vi "PSLDAQ_Read.vi"(4 "Handle In":T1) -> (0 "Int16 Ch2 Data":i16[](array[numeric]), 1 "# Read":i32, 2 "CH2 Data":dbl[](graph), 3 "Int16 Ch1 Data":i16[](array[numeric]), 5 "CH1 Data":dbl[](graph))   [LabVIEW 2010]
doc: "1. 설명\n a. 획득된 데이터를 읽음\n\n2. 기능\n a. PSL-DAQ 장치에서 획득된 2채널의 데이터를 읽음\n \n3. 터미널\n a. 터미널 입력\n ○ Handle In : 장치 핸들\n \n b. 터미널 출력\n ○ Chn Data(n=1~2) : 2채널의 각 채널별 double형 배열 데이터\n ○ Int16 Chn Data(n=1~2) : 2채널의 각 채널별 16bit 부호있는 정수형 배열 데이터\n - PSL-DAQ장치의 ADC 값임. 필요시 데이터 수신 오류 등을 판단할 때 사용 \n ○ #Read : 배열 데이터의 배열의 크기. VI가 호출될 때 읽은 데이터 샘플 수를 의미\n\n4. 주의\n a. PSL DAQ 장치와 통신 연결된 경우에 정상적으로 동작함.\n b. PSLDAQ_AcquireStart 함수가 먼저 호출되어야 함."
uses:
  PSLDAQ_Dll.dll
panel:
  out "# Total Read Num":i32
  # "PSLDAQ_Read\n\n1. 설명\n  a. 획득된 데이터를 읽음\n\n2. 기능\n  a. PSL-DAQ 장치에서 획득된 2채널의 데이터를 읽음\n      \n3. 터미널\n  a. 터미널 입력\n     ○ Handle In : 장치 핸들\n \n  b. 터미널 출력\n     ○ Chn Data(n=1~2) : 2채널의 각 채널별 double형 배열 데이터\n     ○ Int16 Chn Data(n=1~2) : 2채널의 각 채널별 16bit 부호있는 정수형 배열 데이터\n         - PSL-DAQ장치의 ADC 값임. 필요시 데이터 수신 오류 등을 판단할 때 사용 \n     ○ #Read : 배열 데이터의 배열의 크기. VI가 호출될 때 읽은 데이터 샘플 수를 의미\n\n4. 주의\n  a. PSL DAQ 장치와 통신 연결된 경우에 정상적으로 동작함.\n  b. PSLDAQ_AcquireStart 함수가 먼저 호출되어야 함."
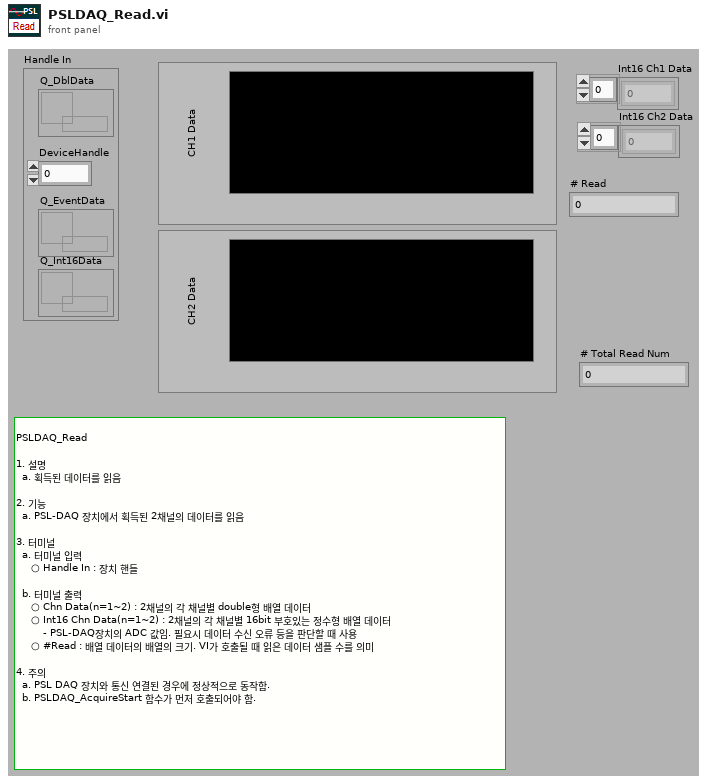
[diagram p1: front panel]
types:
  T1 = cluster{"Q_DblData":refnum<queue>, "DeviceHandle":u32, "Q_EventData":refnum<queue>, "Q_Int16Data":refnum<queue>}
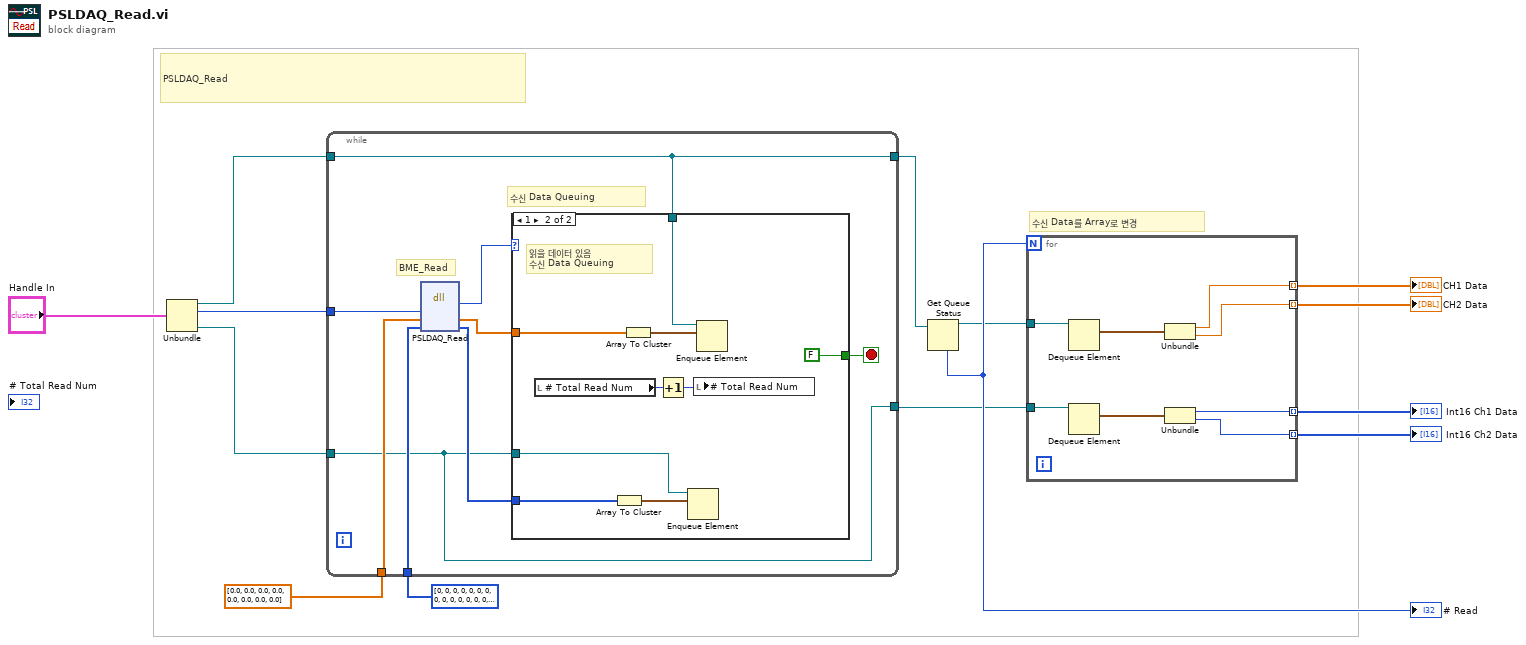
[diagram p0: block diagram]
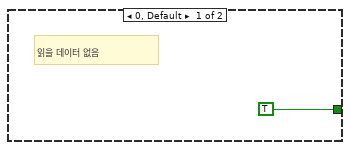
[diagram p2: hidden frame]
diagram:
  # "수신 Data를 Array로 변경"
  # "PSLDAQ_Read"
  n1 = Unbundle("Handle In") -> ("Q_DblData"=w11:refnum<queue>, "DeviceHandle"=w14:u32, "Q_Int16Data"=w5:refnum<queue>)  [unwired: 1 out]
  n2 = while {
    tunnel: w11 -> [w23]
    tunnel: w14 -> [w19]
    tunnel: i16[] [0, 0, 0, 0, 0, 0, 0, 0, 0, 0, 0, 0, 0, 0, 0, 0, 0, 0, 0, 0, 0, 0, 0, 0] -> [w21]
    tunnel: dbl[] [0.0, 0.0, 0.0, 0.0, 0.0, 0.0, 0.0, 0.0] -> [w20]
    tunnel: [w23] -> w7
    tunnel: w5 -> [w15]
    tunnel: [w15] -> w4
    stop <- w22 stop-if-true
    # "BME_Read"
    # "수신 Data Queuing"
    n3 = dll-call lib="D:/PSL-DAQ LabVIEW Library/PSLDAQ_Dll.dll" fn="PSLDAQ_Read"("DeviceHandle"=w19, "DblData"=w20, "Int16Data"=w21) -> ("return type"=w18:u8, "DblData"=w17:dbl[], "Int16Data"=w16:i16[])  [unwired: 4 in, 2 out]
    n4 = case shown="1" w18 {
      tunnel: [TRUE FALSE] -> w22
      tunnel: w23 -> [_ w32]
      tunnel: w17 -> [_ w30]
      tunnel: w16 -> [_ w26]
      tunnel: w15 -> [_ w25]
      frame 0, Default {
        # "읽을 데이터 없음"
      }
      frame 1 {
        # "읽을 데이터 있음\n수신 Data Queuing"
        n5 = local read "# Total Read Num"() -> (w28:i32)
        n6 = Array To Cluster(array=w26) -> (cluster=w27:cluster{"Int16Data[0]":i16, "Int16Data[1]":i16})
        n7 = Array To Cluster(array=w30) -> (cluster=w31:cluster{"DblData[0]":dbl, "DblData[1]":dbl})
        n8 = Increment(x=w28) -> (x+1=w29:i32)
        n9 = Enqueue Element(queue=w25, element=w27) -> ()  [unwired: 2 in, 3 out]
        n10 = local write "# Total Read Num"(w29) -> ()
        n11 = Enqueue Element(queue=w32, element=w31) -> ()  [unwired: 2 in, 3 out]
      }
    }
  }
  n12 = Get Queue Status(queue=w7) -> (queue out=w8:refnum<queue>, # elements in queue=w10:i32)  [unwired: 2 in, 6 out]
  "# Read" <- w10
  n13 = for {
    N: w10 -> [_]
    tunnel: w8 -> [w41]
    tunnel: [w40] -> w9 mode=indexing
    tunnel: [w39] -> w3 mode=indexing
    tunnel: w4 -> [w36]
    tunnel: [w35] -> w2 mode=indexing
    tunnel: [w34] -> w1 mode=indexing
    n14 = Dequeue Element(queue=w41) -> (element=w38:cluster{"[0]":dbl, "[1]":dbl})  [unwired: 2 in, 3 out]
    n15 = Dequeue Element(queue=w36) -> (element=w37:cluster{"[0]":i16, "[1]":i16})  [unwired: 2 in, 3 out]
    n16 = Unbundle(w38) -> ("[0]"=w40:dbl, "[1]"=w39:dbl)
    n17 = Unbundle(w37) -> ("[0]"=w35:i16, "[1]"=w34:i16)
  }
  "CH1 Data" <- w9
  "CH2 Data" <- w3
  "Int16 Ch1 Data" <- w2
  "Int16 Ch2 Data" <- w1
